vi "Map Type.vi"(8 "error in (no error)":errorcluster, 10 "Type":variant, 11 "Sqlite Database Manager in":refnum<class "Sqlite Database Manager.lvclass">) -> (0 "error out":errorcluster, 1 "Mapped Type":string, 3 "Sqlite Database Manager out":refnum<class "Sqlite Database Manager.lvclass">)   [LabVIEW 2019, in "HierDAL Library.lvlib" / "Database.lvlib" / "Sqlite Database Manager.lvclass"]
doc: "Maps a G type to its corresponding database type using a provided mapping.\n\n<b>Type</b> - The G type to map to a database type (e.g., I32, DBL).\n<b>Mapped Type</b> - The corresponding database type as a string."
uses:
  Sqlite Database Manager.lvclass
  <vilib>/Utility/Data Type/NI_Data Type.lvlib
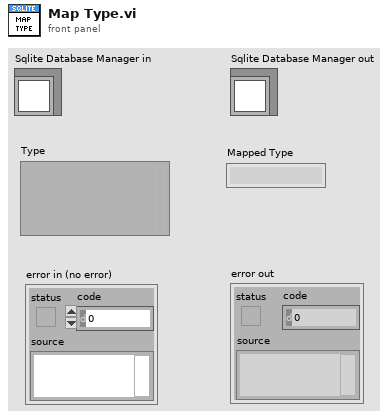
[diagram p1: front panel]
types:
  T1 = typedef "NI_Data Type.lvlib/Data Type.ctl" = enum8{"Invalid Type", "Void", "I8", "I16", "I32", "I64", "U8", "U16", "U32", "U64", "Single Float", "Double Float", "Extended Float", "Single Complex", "Double Complex", "Extended Complex", "Enum U8", "Enum U16", "Enum U32", "Enum U64", "Single Float With Unit", "Double Float With Unit", "Extended Float With Unit", "Single Complex with Unit", "Double Complex with Unit", "Extended Complex with Unit", "Boolean", "String", "Path", "Picture", "Tag", "Array", "Cluster", "Variant", "LV Variant", "Waveform", "Timestamp", "Digital Waveform", "Digital Data", "ExpressData", "Refnum", "External Data", "VI", "Poly VI", "LabVIEW Class Instance", "Fixed Point", "Set Collection", "Map Collection"}
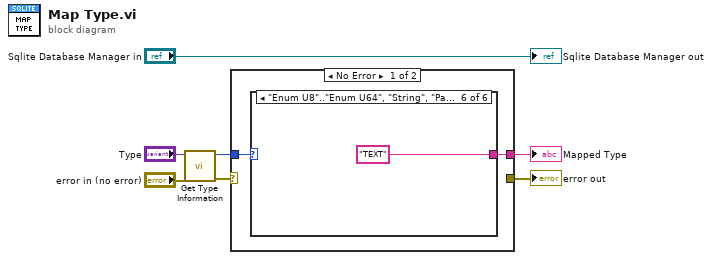
[diagram p0: block diagram]
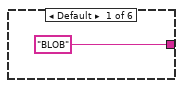
[diagram p2: hidden frame]
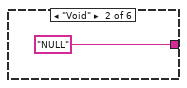
[diagram p3: hidden frame]
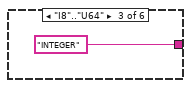
[diagram p4: hidden frame]
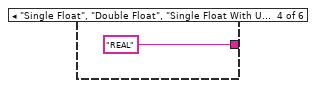
[diagram p5: hidden frame]
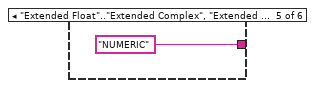
[diagram p6: hidden frame]
diagram:
  n1 = call <vilib>:"Get Type Information.vi"("error in (no error)"="error in (no error)", "variant"="Type") -> ("error out"=w4:errorcluster, "type"=w3:T1)  [unwired: 5 in, 3 out]
  n2 = case shown="No Error" w4 {
    selector: w4 -> [_ w16]
    tunnel: w3 -> [w9 _]
    tunnel: [_ w16] -> w2
    tunnel: [w8 _] -> w1
    frame No Error {
      n3 = case shown="\"Enum U8\"..\"Enum U64\", \"String\", \"Path\", \"Timestamp\"" w9 {
        tunnel: ["BLOB" "NULL" "INTEGER" "REAL" "NUMERIC" "TEXT"] -> w8
        frame Default {
        }
        frame "Void" {
        }
        frame "I8".."U64" {
        }
        frame "Single Float", "Double Float", "Single Float With Unit", "Double Float With Unit" {
        }
        frame "Extended Float".."Extended Complex", "Extended Float With Unit".."Boolean", "Refnum" {
        }
        frame "Enum U8".."Enum U64", "String", "Path", "Timestamp" {
        }
      }
    }
    frame Error {
    }
  }
  "error out" <- w2
  "Mapped Type" <- w1
  "Sqlite Database Manager out" <- "Sqlite Database Manager in"
